vi "Set Running.vi"(8 "error in (no error)":errorcluster, 10 "Running":bool, 11 "2DArrayManager in":refnum<class "2DArrayManager.lvclass">) -> (0 "error out":errorcluster, 3 "2DArrayManager out":refnum<class "2DArrayManager.lvclass">)   [LabVIEW 2020, in "OOPanel.lvlib" / "2DArrayManager.lvclass"]
uses:
  2DArrayManager.lvclass
  2DArrayManager.lvclass/2DArrayManager.ctl
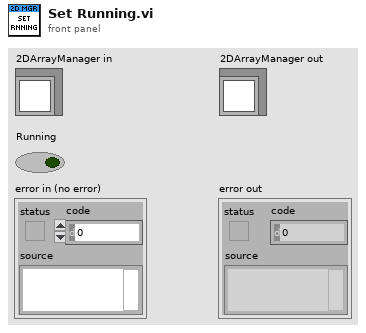
[diagram p1: front panel]
types:
  T1 = typedef "OOPanel.lvlib/2DArrayManager.lvclass/State Ref.ctl" = cluster{"Running":bool, "Borders":bool, "Total Height":dbl, "Background":u32, "V Scroll":bool, "H Scroll":bool}
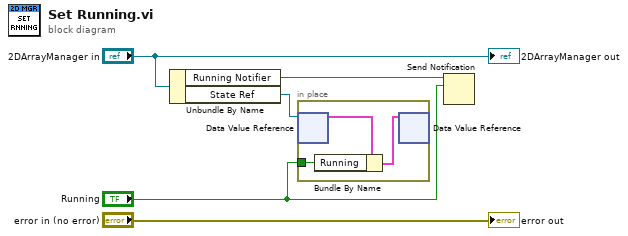
[diagram p0: block diagram]
diagram:
  n1 = Unbundle By Name("2DArrayManager in") -> ("Running Notifier"=w3:refnum<notifier>, "State Ref"=w4:refnum<data-value>)
  n2 = in-place {
    in-place-border: "Running" -> [w6]
    n3 = in-place-dvr #1(w4) -> (w8:T1)  [unwired: 1 out]
    n4 = Bundle By Name(cluster=w8, "Running"=w6) -> (w7:T1)
    n5 = in-place-dvr #1(w7) -> ()  [unwired: 2 out]
  }
  n6 = Send Notification(notification="Running", notifier=w3) -> ()  [unwired: 1 in, 2 out]
  "error out" <- "error in (no error)"
  "2DArrayManager out" <- "2DArrayManager in"
